vi "Page Demo.vi"() -> ()   [LabVIEW 2018, in "Page.lvlib"]
uses:
  Page.lvlib
  Page Action.ctl
  Page Refnums.ctl
  Page Mouse.ctl
  <vilib>/Utility/miscctls.llb/LVPoint32TypeDef.ctl
  Page Test.vi
  Exit/Exit.lvlib
panel:
  in  "Select":bool
  out "Picture":picture
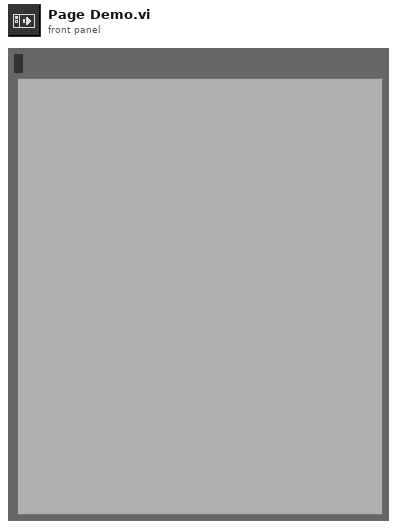
[diagram p1: front panel]
types:
  T1 = typedef "Page.lvlib/Page Action.ctl" = enum8{"noop", "new", "init", "close", "page_change", "page_hover", "render", "page_caption", "page_insert", "page_add", "start", "resize", "theme_change", "hide"}
  T2 = typedef "Page.lvlib/Page Refnums.ctl" = cluster{"VI Refnum":refnum<vi>, "Sub Panel":refnum<vi>, "Picture":refnum<vi>}
  T3 = typedef "Page.lvlib/Page Mouse.ctl" = cluster{"Horizontal":i32, "Vertical":i32, "Button":u16, "Shift":bool, "Ctrl":bool, "Alt":bool, "Double Click":bool}
  T4 = typedef "LVPoint32TypeDef.ctl" = cluster{"Horizontal":i32, "Vertical":i32}
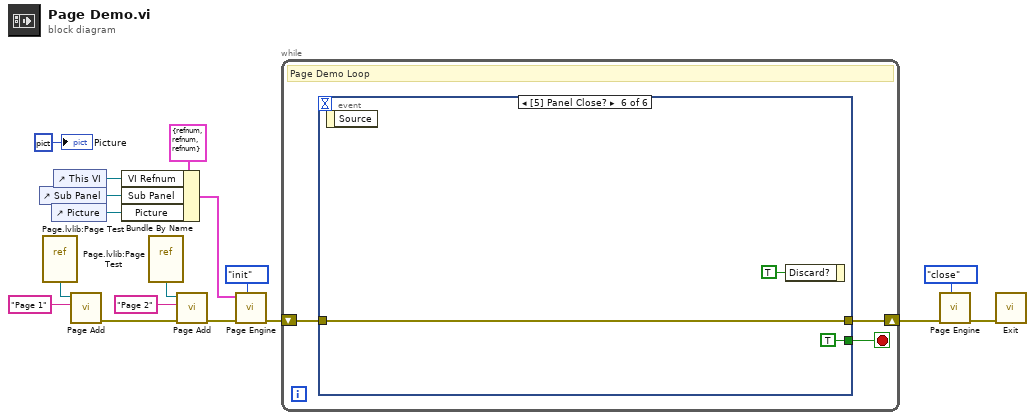
[diagram p0: block diagram]
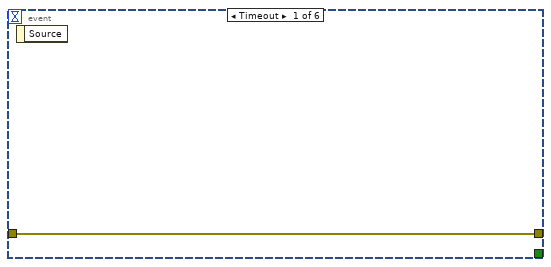
[diagram p2: hidden frame]
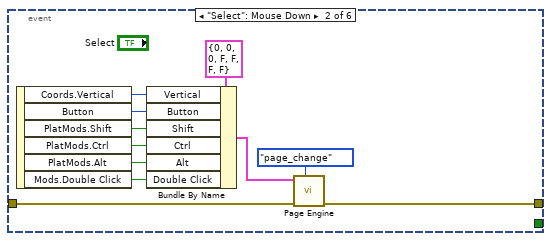
[diagram p3: hidden frame]
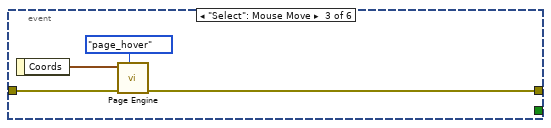
[diagram p4: hidden frame]
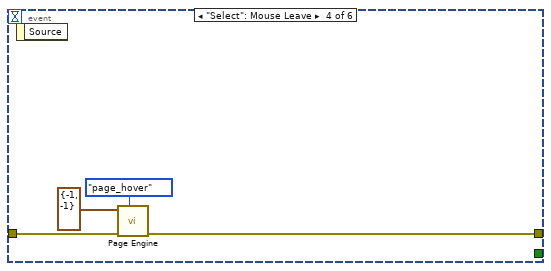
[diagram p5: hidden frame]
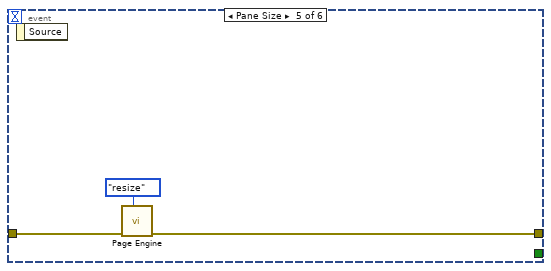
[diagram p6: hidden frame]
diagram:
  n1 = control-ref of="Sub Panel"() -> (w14:refnum<vi>)
  n2 = vi-ref "Page.lvlib:Page Test.vi"() -> (w9:refnum<vi>)
  n3 = control-ref of="Picture"() -> (w13:refnum<vi>)
  n4 = control-ref of="This VI"() -> (w15:refnum<vi>)
  n5 = call "Page Add.vi"("Caption"="Page 1", "VI Refnum"=w9) -> ("error out"=w5:errorcluster)  [unwired: 9 in]
  n6 = Bundle By Name(cluster=T2 {"VI Refnum"=refnum, "Sub Panel"=refnum, "Picture"=refnum} ("Refnums"), "VI Refnum"=w15, "Sub Panel"=w14, "Picture"=w13) -> (w12:T2)
  n7 = vi-ref "Page.lvlib:Page Test.vi"() -> (w6:refnum<vi>)
  n8 = call "Page Add.vi"("error in (no error)"=w5, "Caption"="Page 2", "VI Refnum"=w6) -> ("error out"=w4:errorcluster)  [unwired: 8 in]
  n9 = call "Page Engine.vi"("Action"=Page_Action."init", "error in (no error)"=w4, "Data in"=w12) -> ("error out"=w11:errorcluster)  [unwired: 7 in, 1 out]
  n10 = while {
    shift-right: [w18] -> w2
    shift-left: w11 -> [w19]
    stop <- w20 stop-if-true
    # "Page Demo Loop"
    n11 = event shown="[5] Panel Close?" {
      selector: _ -> [_ _ _ _ _ _]
      dyn-events: _ -> [_ _ _ _ _ _]
      timeout: _ -> [_ _ _ _ _ _]
      tunnel: [_ _ _ _ _ TRUE ("T button?")] -> w20
      tunnel: w19 -> [w21 w31 w35 w39 w42 w45]
      tunnel: [w21 w30 w34 w38 w41 w45] -> w18
      event Timeout {
        n12 = event-data() -> ()  [unwired: 1 in, 1 out]
      }
      event "Select": Mouse Down {
        n13 = event-data() -> ("Coords.Vertical"=w27:i32, "Button"=w26:u16, "PlatMods.Shift"=w25:bool, "PlatMods.Ctrl"=w24:bool, "PlatMods.Alt"=w23:bool, "Mods.Double Click"=w22:bool)  [unwired: 1 in]
        n14 = Bundle By Name(cluster=T3 {"Horizontal"=0, "Vertical"=0, "Button"=0, "Shift"=FALSE, "Ctrl"=FALSE, "Alt"=FALSE, "Double Click"=FALSE} ("Page Mouse"), "Vertical"=w27, "Button"=w26, "Shift"=w25, "Ctrl"=w24, "Alt"=w23, "Double Click"=w22) -> (w28:T3)
        n15 = call "Page Engine.vi"("Action"=Page_Action."page_change", "error in (no error)"=w31, "Data in"=w28) -> ("error out"=w30:errorcluster)  [unwired: 7 in, 1 out]
      }
      event "Select": Mouse Move {
        n16 = event-data() -> ("Coords"=w33:T4)  [unwired: 1 in]
        n17 = call "Page Engine.vi"("Action"=Page_Action."page_hover", "error in (no error)"=w35, "Data in"=w33) -> ("error out"=w34:errorcluster)  [unwired: 7 in, 1 out]
      }
      event "Select": Mouse Leave {
        n18 = event-data() -> ()  [unwired: 1 in, 1 out]
        n19 = call "Page Engine.vi"("Action"=Page_Action."page_hover", "error in (no error)"=w39, "Data in"=T4 {"Horizontal"=-1, "Vertical"=-1} ("Coords")) -> ("error out"=w38:errorcluster)  [unwired: 7 in, 1 out]
      }
      event Pane Size {
        n20 = event-data() -> ()  [unwired: 1 in, 1 out]
        n21 = call "Page Engine.vi"("Action"=Page_Action."resize", "error in (no error)"=w42) -> ("error out"=w41:errorcluster)  [unwired: 8 in, 1 out]
      }
      event Panel Close? {
        n22 = event-data() -> ()  [unwired: 1 in, 1 out]
        n23 = event-data("Discard?"=TRUE) -> ()  [unwired: 1 in, 1 out]
      }
    }
  }
  n24 = call "Page Engine.vi"("Action"=Page_Action."close", "error in (no error)"=w2) -> ("error out"=w1:errorcluster)  [unwired: 8 in, 1 out]
  n25 = call "Exit.vi"("error in (no error)"=w1) -> ()  [unwired: 10 in, 1 out]
  "Picture" <- picture data[5B] ("Picture")
